vi "Read_Write_Local_table_Quick.vi"(3 "Mode":T1, 4 "String Values In":string[](array[string]), 5 "Ch names In":string[](array[string])) -> (0 "Numeric Values Out":dbl[](array[numeric]), 1 "String Values Out":string[](array[string]), 2 "Ch Names Out":string[](array[string]))   [LabVIEW 2015]
uses:
  ADAM Controls/Quick_local_ADAM_Table.ctl
  ADAM Controls/Channel_names.ctl
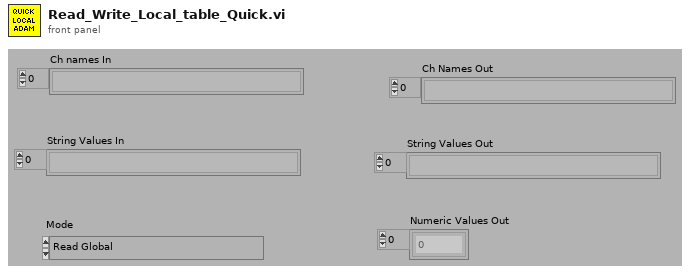
[diagram p1: front panel]
types:
  T1 = typedef "Quick_local_ADAM_Table.ctl" = enum16{"Read Global", "Load Global From ADAM Table", "Write Global"}
  T2 = typedef "Channel_names.ctl" = enum16{"Active Only", "Active + Off", "All Channels"}
  T3 = typedef "Ch_description_ADAM.ctl" = cluster{"Ch Name":string, "Type":T4, "Function":T5, "Ch State":T6, "Calibration type":T7, "A":dbl, "B":dbl, "C":dbl, "D":dbl, "Comments":string, "Address":T8, "String":string, "Duty":u16}
  T4 = typedef "Module_type_ADAM.ctl" = string
  T5 = typedef "Function_ADAM.ctl" = enum16{"Analogue Input", "Digital Input", "Event counter", "Event rate", "Analogue Output", "Digital Output", "Relay Output"}
  T6 = typedef "Channel_State.ctl" = enum16{"On", "Off", "Always On", "Always Off"}
  T7 = typedef "Calib_type_ADAM.ctl" = enum16{"Raw", "Bx + A", "Cx^2 + Bx + A", "Dx^3 + Cx^2 + Bx + A", "In Band", "Hi-Tec Q", "Hi-Tec M_dot", "Text"}
  T8 = typedef "Address.ctl" = cluster{"Main":i32, "Ch.":i32, "Sub":i32, "Port Name":string}
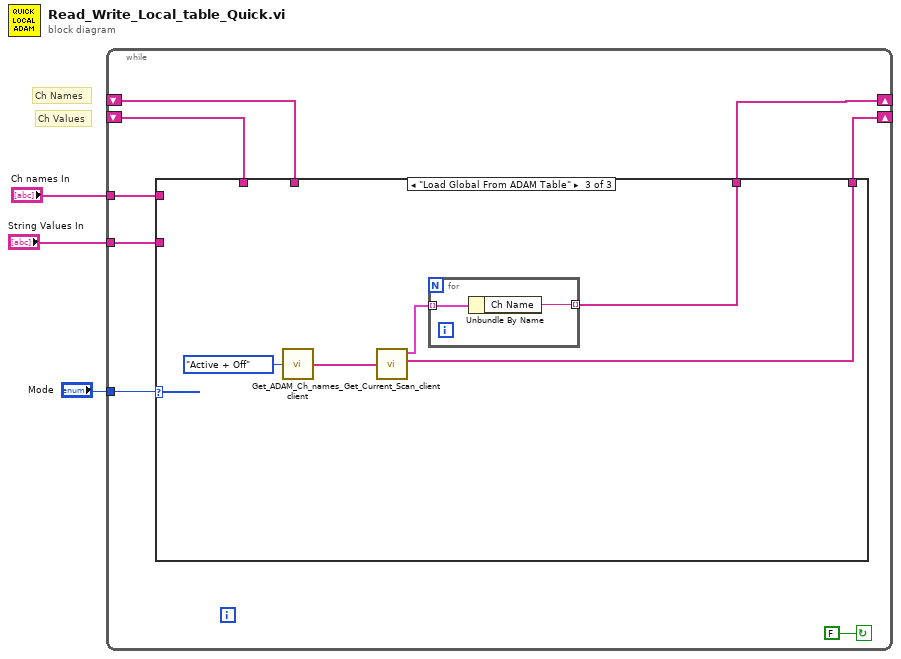
[diagram p0: block diagram]
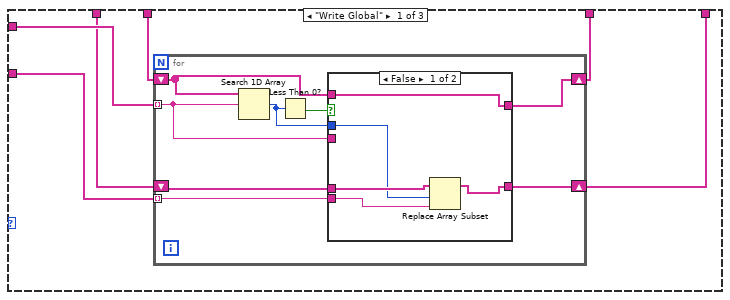
[diagram p2: hidden frame]
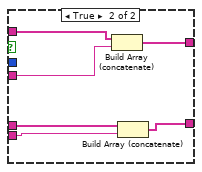
[diagram p3: hidden frame]
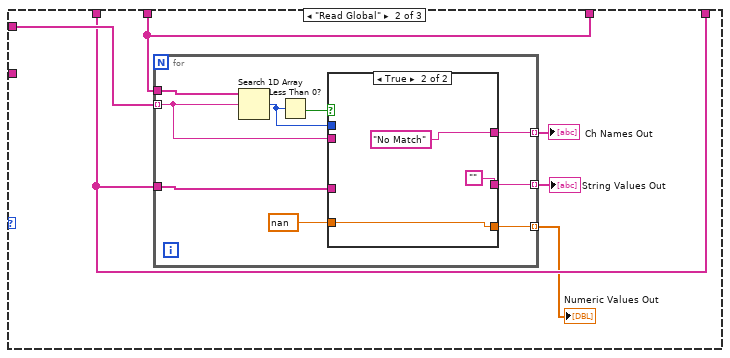
[diagram p4: hidden frame]
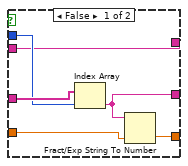
[diagram p5: hidden frame]
diagram:
  # "Ch Values"
  # "Ch Names"
  n1 = while {
    shift-left: _ -> [w7]
    shift-right: [w8] -> _
    shift-left: _ -> [w10]
    shift-right: [w9] -> _
    tunnel: "Mode" -> [w11]
    tunnel: "Ch names In" -> [w6]
    tunnel: "String Values In" -> [w5]
    stop <- FALSE continue-if-true
    n2 = case shown="\"Load Global From ADAM Table\"" w11 {
      tunnel: w6 -> [w17 w42 _]
      tunnel: w10 -> [w16 w41 _]
      tunnel: [w15 w41 w61] -> w9
      tunnel: w7 -> [w14 w40 _]
      tunnel: w5 -> [w13 _ _]
      tunnel: [w12 w40 w63] -> w8
      frame "Write Global" {
        n3 = for {
          tunnel: w17 -> [w23] mode=indexing
          shift-right: [w22] -> w15
          shift-left: w16 -> [w24]
          shift-right: [w19] -> w12
          shift-left: w14 -> [w21]
          tunnel: w13 -> [w20] mode=indexing
          n4 = Search 1D Array(1D array=w24, element=w23) -> (index of element=w18:i32)  [unwired: 1 in]
          n5 = Less Than 0?(x=w18) -> (x < 0?=w25:bool)
          n6 = case shown="False" w25 {
            tunnel: w24 -> [w26 w36]
            tunnel: w23 -> [_ w35]
            tunnel: [w26 w34] -> w22
            tunnel: w21 -> [w30 w33]
            tunnel: w20 -> [w28 w32]
            tunnel: [w27 w31] -> w19
            tunnel: w18 -> [w29 _]
            frame False {
              n7 = Replace Array Subset(array=w30, new element=w28, index=w29) -> (w27:string[])
            }
            frame True {
              n8 = Build Array (concatenate)(w36, w35) -> (w34:string[])
              n9 = Build Array (concatenate)(w33, w32) -> (w31:string[])
            }
          }
        }
      }
      frame "Read Global" {
        n10 = for {
          tunnel: w42 -> [w50] mode=indexing
          tunnel: w40 -> [w48]
          tunnel: w41 -> [w47]
          tunnel: [w46] -> w39 mode=indexing
          tunnel: [w45] -> w38 mode=indexing
          tunnel: [w44] -> w37 mode=indexing
          n11 = Search 1D Array(1D array=w47, element=w50) -> (index of element=w49:i32)  [unwired: 1 in]
          n12 = Less Than 0?(x=w49) -> (x < 0?=w51:bool)
          n13 = case shown="True" w51 {
            tunnel: w50 -> [w55 _]
            tunnel: w48 -> [w57 _]
            tunnel: w49 -> [w56 _]
            tunnel: [w55 "No Match"] -> w46
            tunnel: [w54 ""] -> w45
            tunnel: [w53 w58] -> w44
            tunnel: nan ("default (0 DBL)") -> [w52 w58]
            frame False {
              n14 = Index Array(array=w57, index=w56) -> (element=w54:string)
              n15 = Fract/Exp String To Number(string=w54, default (0 dbl)=w52) -> (number=w53:dbl)  [unwired: 2 in, 1 out]
            }
            frame True {
            }
          }
        }
        "Ch Names Out" <- w39
        "String Values Out" <- w38
        "Numeric Values Out" <- w37
      }
      frame "Load Global From ADAM Table" {
        n16 = call "Get_ADAM_Ch_names_client.vi"("Channel names set"=Channel_names."Active + Off") -> ("Ch names"=w64:string[])
        n17 = call "Get_Current_Scan_client.vi"("ADAM Ch Names"=w64) -> ("Ch Description Array"=w62:T3[], "String values"=w63:string[])  [unwired: 1 in, 1 out]
        n18 = for {
          tunnel: w62 -> [w67] mode=indexing
          tunnel: [w66] -> w61 mode=indexing
          n19 = Unbundle By Name(w67) -> ("Ch Name"=w66:string)
        }
      }
    }
  }
